vi "GoToTarget.vi"(8 "error in (no error)":errorcluster, 9 "Ball":refnum<class "Ball.lvclass">, 10 "Robot":refnum<class "Robot.lvclass">, 11 "object in":refnum<class "GoToSkill_v2.lvclass">) -> (0 "error out":errorcluster, 2 "Robot out":refnum<class "Robot.lvclass">, 3 "object out":refnum<class "GoToSkill_v2.lvclass">)   [LabVIEW 2023, in "GoToSkill_v2.lvclass"]
uses:
  GoToSkill_v2.lvclass
  Robot_class/Robot.lvclass
  Ball_class/Ball.lvclass
  C:/Users/ebert/Documents/codes/SSL/repo/SSL_AI/Object_class/Object.lvclass
  Object_class/Object.lvclass/Object.ctl
  Object_class/Read position(x,y).vi
  Zone_class/Zone.lvclass
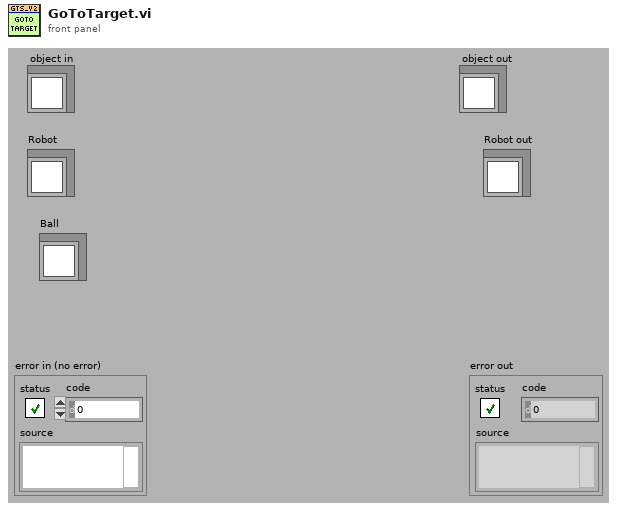
[diagram p1: front panel]
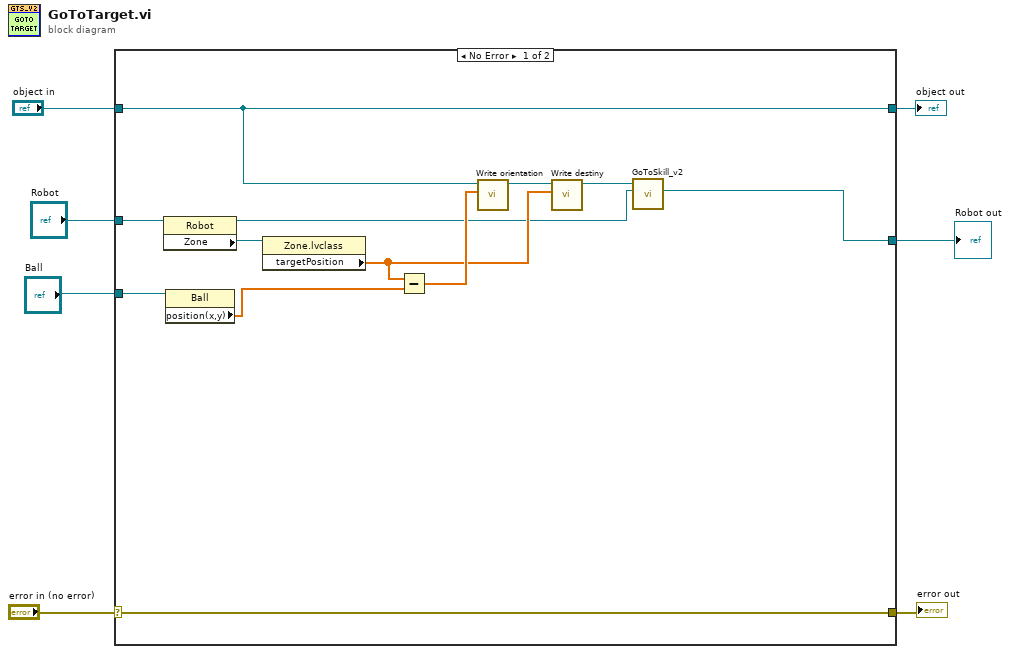
[diagram p0: block diagram]
diagram:
  n1 = case shown="No Error" "error in (no error)" {
    selector: "error in (no error)" -> [w19 w22]
    tunnel: [w19 w22] -> w6
    tunnel: [w18 w21] -> w4
    tunnel: "object in" -> [w18 w21]
    tunnel: "Ball" -> [w15 _]
    tunnel: "Robot" -> [w14 w20]
    tunnel: [w8 w20] -> w1
    frame No Error {
      n2 = property class="Robot"(reference=w14) -> (reference out=w9:refnum<class "Robot.lvclass">, "Zone"=w13:refnum<class "Zone.lvclass">)  [unwired: 1 in, 1 out]
      n3 = property class="Ball"(reference=w15) -> ("position(x,y)"=w12:dbl[])  [unwired: 1 in, 2 out]
      n4 = property class="Zone.lvclass"(reference=w13) -> ("targetPosition"=w10:dbl[])  [unwired: 1 in, 2 out]
      n5 = Subtract(x=w10, y=w12) -> (x-y=w11:dbl[])
      n6 = call-dynamic "Write orientation.vi"("orientation"=w11, "GoToSkill_v2 in"=w18) -> ("GoToSkill_v2 out"=w17:refnum<class "GoToSkill_v2.lvclass">)  [unwired: 8 in, 1 out]
      n7 = call-dynamic "Write destiny.vi"("destiny"=w10, "GoToSkill_v2 in"=w17) -> ("GoToSkill_v2 out"=w16:refnum<class "GoToSkill_v2.lvclass">)  [unwired: 8 in, 1 out]
      n8 = call-dynamic "GoToSkill_v2.vi"("Robot"=w9, "object in"=w16) -> ("Robot out"=w8:refnum<class "Robot.lvclass">)  [unwired: 7 in, 2 out]
    }
    frame Error {
    }
  }
  "error out" <- w6
  "object out" <- w4
  "Robot out" <- w1
